vi "SwerveCalculations.vi"() -> ()   [LabVIEW 2016]
uses:
  Robot Global Data.vi
panel:
  in  "Auto Enabled":bool
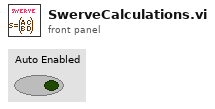
[diagram p1: front panel]
types:
  T1 = enum16{"X-axis", "Y-axis", "LTrigger", "RTrigger", "R-Xaxis", "R-Yaxis"}
  T2 = enum16{"A-but", "B-but", "Xbut", "Y-but", "L-but", "R_but"}
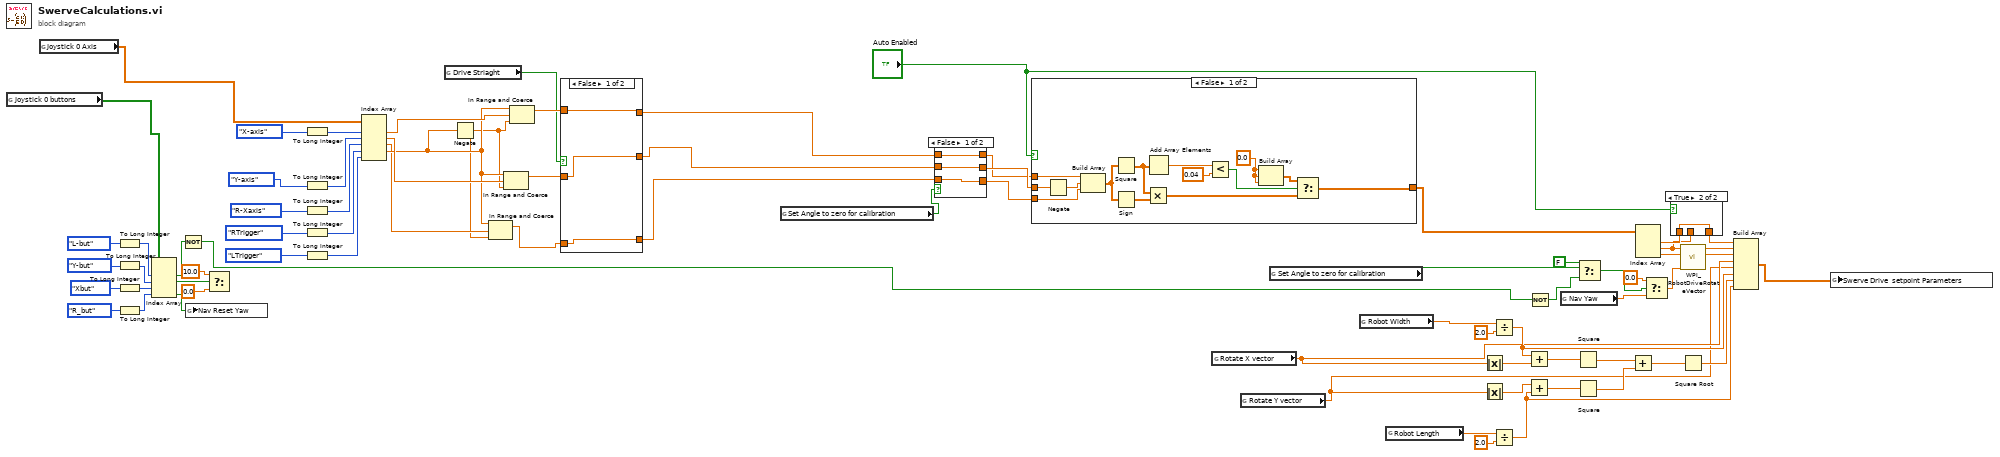
[diagram p0: block diagram]
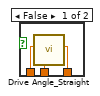
[diagram p2: hidden frame]
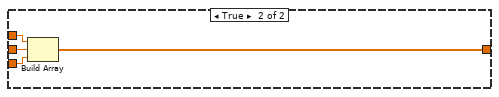
[diagram p3: hidden frame]
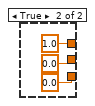
[diagram p4: hidden frame]
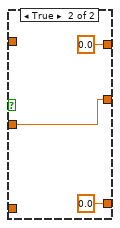
[diagram p5: hidden frame]
diagram:
  n1 = global read "Robot Global Data.vi" "Joystick 0 buttons"() -> (w46:bool[])
  n2 = global read "Robot Global Data.vi" "Joystick 0 Axis"() -> (w47:dbl[])
  n3 = To Long Integer(number=T2."L-but") -> (32bit integer=w70:i32)
  n4 = To Long Integer(number=T2."Y-but") -> (32bit integer=w69:i32)
  n5 = To Long Integer(number=T2."Xbut") -> (32bit integer=w68:i32)
  n6 = To Long Integer(number=T2."R_but") -> (32bit integer=w67:i32)
  n7 = Index Array(array=w46, index #1=w70, index #2=w69, index #3=w68, index #4=w67) -> (element #1=w62:bool, element #2=w66:bool, element #4=w63:bool)  [unwired: 1 out]
  n8 = Not(x=w62) -> (.not. x?=w3:bool)
  n9 = global write "Robot Global Data.vi" "Nav Reset Yaw"(w63) -> ()
  n10 = Select(t=10.0, s=w66, f=0.0) -> ()  [unwired: 1 out]
  n11 = To Long Integer(number=T1."X-axis") -> (32bit integer=w59:i32)
  n12 = To Long Integer(number=T1."Y-axis") -> (32bit integer=w58:i32)
  n13 = To Long Integer(number=T1."R-Xaxis") -> (32bit integer=w57:i32)
  n14 = To Long Integer(number=T1."RTrigger") -> (32bit integer=w55:i32)
  n15 = To Long Integer(number=T1."LTrigger") -> (32bit integer=w53:i32)
  n16 = Index Array(array=w47, index #1=w59, index #2=w58, index #3=w57, index #4=w55, index #5=w53) -> (element #1=w52:dbl, element #2=w51:dbl, element #3=w49:dbl, element #4=w50:dbl)  [unwired: 1 out]
  n17 = global read "Robot Global Data.vi" "Drive Striaght"() -> (w41:bool)
  n18 = Negate(x=w50) -> (-x=w45:dbl)
  n19 = In Range and Coerce(upper limit=w50, x=w49, lower limit=w45) -> (coerced(x)=w44:dbl)  [unwired: 1 out]
  n20 = In Range and Coerce(upper limit=w50, x=w51, lower limit=w45) -> (coerced(x)=w43:dbl)  [unwired: 1 out]
  n21 = In Range and Coerce(upper limit=w50, x=w52, lower limit=w45) -> (coerced(x)=w42:dbl)  [unwired: 1 out]
  n22 = case shown="False" w41 {
    tunnel: w44 -> [w75 _]
    tunnel: [w75 0.0 ("Numeric")] -> w37
    tunnel: w43 -> [w76 w78]
    tunnel: [w76 w78] -> w38
    tunnel: w42 -> [w77 _]
    tunnel: [w77 0.0 ("Numeric")] -> w39
    frame False {
    }
    frame True {
    }
  }
  n23 = global read "Robot Global Data.vi" "Set Angle to zero for calibration"() -> (w40:bool)
  n24 = case shown="False" w40 {
    tunnel: w38 -> [w83 _]
    tunnel: [w83 0.0 ("Y")] -> w35
    tunnel: w39 -> [w82 _]
    tunnel: [w82 1.0 ("X")] -> w34
    tunnel: w37 -> [w81 _]
    tunnel: [w81 0.0 ("Z")] -> w36
    frame False {
    }
    frame True {
    }
  }
  n25 = case shown="False" "Auto Enabled" {
    tunnel: [w90 w104] -> w5
    tunnel: w36 -> [w89 w103]
    tunnel: w34 -> [w87 w102]
    tunnel: w35 -> [w88 w101]
    frame False {
      w96 = 0.0 ("element")
      n26 = Negate(x=w88) -> (-x=w92:dbl)
      n27 = Build Array(w87, w92, w89) -> (w95:dbl[])
      n28 = Square(x=w95) -> (x^2=w93:dbl[])
      n29 = Sign(1:w95) -> (0:w94:dbl[])
      n30 = Multiply(x=w93, y=w94) -> (x*y=w91:dbl[])
      n31 = Add Array Elements(numeric array=w93) -> (sum=w100:dbl)
      n32 = Less?(x=w100, y=0.04 ("x")) -> (x < y?=w98:bool)
      n33 = Build Array(w96, w96, w96) -> (w97:dbl[])
      n34 = Select(t=w97, s=w98, f=w91) -> (s? t:f=w90:dbl[])
    }
    frame True {
      n35 = Build Array(w102, w101, w103) -> (w104:dbl[])
    }
  }
  n36 = global read "Robot Global Data.vi" "Rotate X vector"() -> (w2:dbl)
  n37 = global read "Robot Global Data.vi" "Rotate Y vector"() -> (w1:dbl)
  n38 = global read "Robot Global Data.vi" "Set Angle to zero for calibration"() -> (w12:bool)
  n39 = global read "Robot Global Data.vi" "Robot Width"() -> (w16:dbl)
  n40 = global read "Robot Global Data.vi" "Robot Length"() -> (w15:dbl)
  n41 = Absolute Value(x=w2) -> (abs(x)=w30:dbl)
  n42 = Absolute Value(x=w1) -> (abs(x)=w28:dbl)
  n43 = Divide(x=w16, y=2.0) -> (x/y=w19:dbl)
  n44 = Divide(x=w15, y=2.0) -> (x/y=w21:dbl)
  n45 = Add(x=w19, y=w30) -> (x+y=w29:dbl)
  n46 = Add(x=w28, y=w21) -> (x+y=w27:dbl)
  n47 = Not(x=w3) -> (.not. x?=w11:bool)
  n48 = global read "Robot Global Data.vi" "Nav Yaw"() -> (w32:dbl)
  n49 = Square(x=w29) -> (x^2=w25:dbl)
  n50 = Square(x=w27) -> (x^2=w26:dbl)
  n51 = Select(t=FALSE, s=w12, f=w11) -> (s? t:f=w10:bool)
  n52 = Add(x=w25, y=w26) -> (x+y=w24:dbl)
  n53 = Index Array(array=w5) -> (element #1=w14:dbl, element #2=w7:dbl, element #3=w8:dbl)  [unwired: 3 in]
  n54 = Select(t=0.0, s=w10, f=w32) -> (s? t:f=w31:dbl)
  n55 = case shown="True" "Auto Enabled" {
    tunnel: w14 -> [w107 w108]
    tunnel: [w106 w108] -> w13
    tunnel: w7 -> [w105 _]
    frame False {
      n56 = call "Drive Angle_Straight.vi"("y input"=w105, "Z axis in"=w107) -> ("Z out"=w106:dbl)  [unwired: 9 in]
    }
    frame True {
    }
  }
  n57 = call <vilib>:"WPI_RobotDriveRotateVector.vi"("Angle"=w31, "X"=w8, "Y"=w7) -> ("X'"=w18:dbl, "Y'"=w17:dbl)  [unwired: 7 out]
  n58 = Square Root(x=w24) -> (sqrt(x)=w20:dbl)
  n59 = Build Array(w13, w17, w18, w2, w1, w19, w20, w21) -> (w4:dbl[])
  n60 = global write "Robot Global Data.vi" "Swerve Drive  setpoint Parameters"(w4) -> ()
